vi "Write Current.vi"(8 "error in":errorcluster, 10 "Current":dbl, 11 "Acopian in":refnum<class "Acopian.lvclass">) -> (0 "error out":errorcluster, 3 "Acopian out":refnum<class "Acopian.lvclass">)   [LabVIEW 2019, in "Acopian.lvlib" / "Acopian.lvclass"]
uses:
  Library/Acopian.lvclass
  C:/Users/Public/Documents/Development/builds/Instruments/PowerSupply.lvlibp/Library/PowerSupply.lvclass
  Library/Acopian.lvclass/Acopian.ctl
  builds/Instruments/PowerSupply.lvlibp/Library/PowerSupply.lvclass
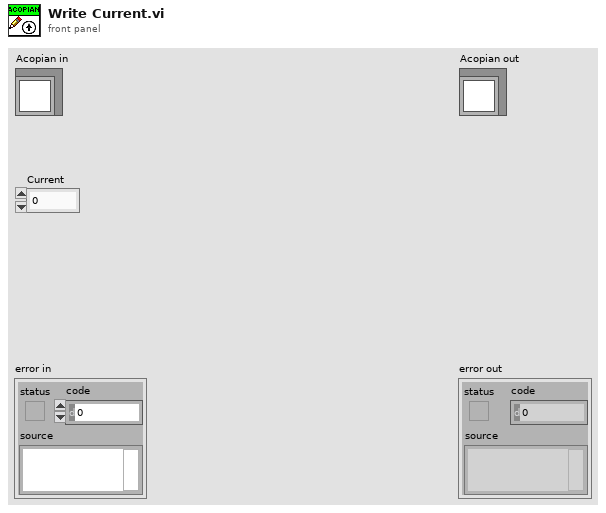
[diagram p1: front panel]
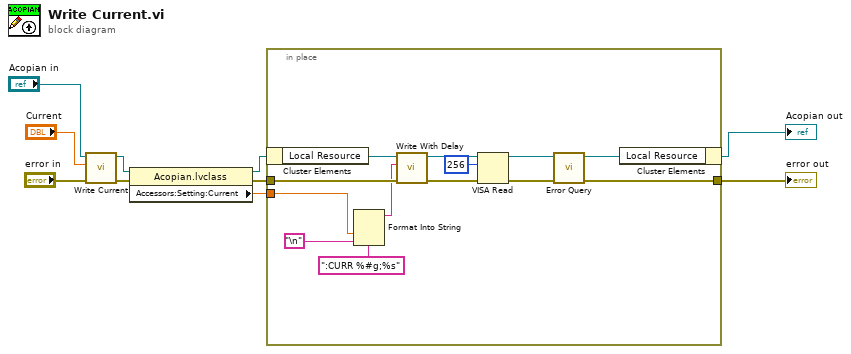
[diagram p0: block diagram]
diagram:
  n1 = call-parent "Write Current.vi"("error in"="error in", "Current"="Current", "PowerSupply in"="Acopian in") -> ("error out"=w7:errorcluster, "PowerSupply out"=w3:refnum<class "Acopian.lvclass">)  [unwired: 7 in]
  n2 = property class="Acopian.lvclass"(reference=w3, error in=w7) -> (reference out=w2:refnum<class "Acopian.lvclass">, error out=w4:errorcluster, "Accessors:Setting:Current"=w1:dbl)
  n3 = in-place {
    in-place-border: w4 -> [w16]
    in-place-border: [w15] -> w5
    in-place-border: w1 -> [w13]
    n4 = in-place-cluster #1(w2) -> ("Local Resource"=w18:refnum<visa-resource-name>)
    n5 = Format Into String(format string=":CURR %#g;%s" ("Current Limit Command"), w13, "\n") -> (resulting string=w12:string)  [unwired: 2 in, 1 out]
    n6 = call "Write With Delay.vi"("error in"=w16, "write buffer"=w12, "VISA resource name"=w18) -> ("error out"=w21:errorcluster, "VISA resource name out"=w20:refnum<visa-resource-name>)  [unwired: 7 in]
    n7 = VISA Read(VISA resource name=w20, byte count=u32 256, error in (no error)=w21) -> (VISA resource name out=w22:refnum<visa-resource-name>, error out=w23:errorcluster)  [unwired: 2 out]
    n8 = call "Error Query.vi"("error in"=w23, "VISA resource in"=w22) -> ("error out"=w15:errorcluster, "VISA resource out"=w17:refnum<visa-resource-name>)  [unwired: 6 in, 2 out]
    n9 = in-place-cluster #1("Local Resource"=w17) -> (→"Acopian out":refnum<class "Acopian.lvclass">)
  }
  "error out" <- w5
